vi "Read Joystick.vi"(8 "error in (no error)":errorcluster, 11 "XBoxController-V in":refnum<class "XBoxController-V.lvclass">) -> (0 "error out":errorcluster, 3 "XBoxController-V out":refnum<class "XBoxController-V.lvclass">)   [LabVIEW 2013, in "VirtualRobot.lvlib" / "XBoxController-V.lvlib" / "XBoxController-V.lvclass"]
uses:
  XBoxController-V.lvclass
  Systems/XBoxController/XboxJoysticks.ctl
  Systems/XBoxController/XBoxController.lvclass
  Systems/XBoxController/XBoxController.lvlib
panel:
  in  "XboxJoysticks":T1 {"RightJoystick"."Right" scale=-1.0..1.0; "RightJoystick"."Forward" scale=-1.0..1.0; "LeftJoystick"."Right" scale=-1.0..1.0; "LeftJoystick"."Forward" scale=-1.0..1.0}
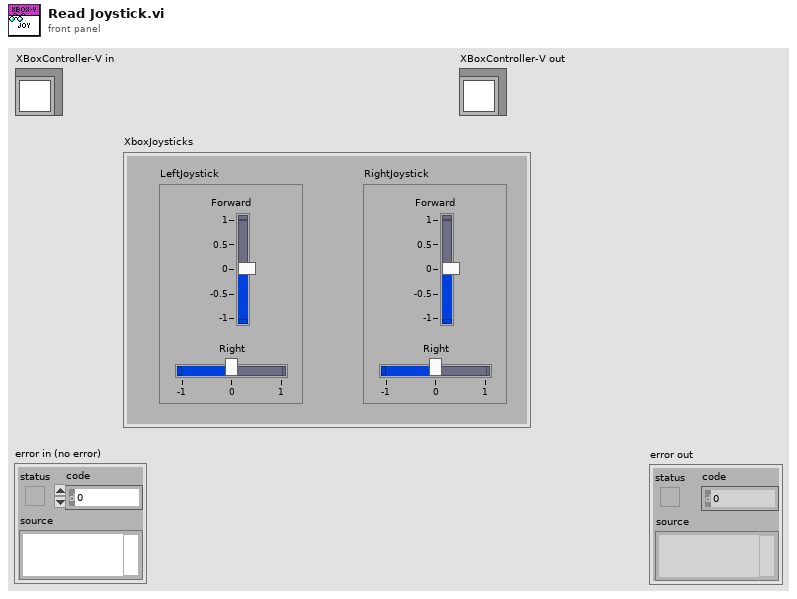
[diagram p1: front panel]
types:
  T1 = typedef "XBoxController.lvlib/XboxJoysticks.ctl" = cluster{"LeftJoystick":cluster{"Forward":dbl, "Right":dbl}, "RightJoystick":cluster{"Forward":dbl, "Right":dbl}}
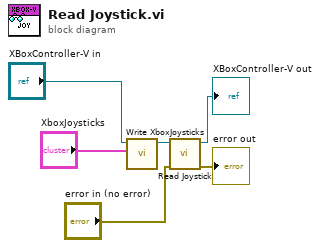
[diagram p0: block diagram]
diagram:
  n1 = call-dynamic "Write XboxJoysticks.vi"("XboxJoysticks"="XboxJoysticks", "XBoxController in"="XBoxController-V in") -> ("XBoxController out"=w2:refnum<class "XBoxController-V.lvclass">)  [unwired: 8 in, 1 out]
  n2 = call-parent "Read Joystick.vi"("error in (no error)"="error in (no error)", "XBoxController in"=w2) -> ("error out"=→"error out":errorcluster, "XBoxController out"=→"XBoxController-V out":refnum<class "XBoxController-V.lvclass">)  [unwired: 8 in]
